vi "Host Save ID Data.vi"(11 "Input RY":T1) -> ()   [LabVIEW 2016]
uses:
  <vilib>/Utility/file.llb/Write Delimited Spreadsheet (string).vi
  <vilib>/Utility/file.llb/Write Delimited Spreadsheet (DBL).vi
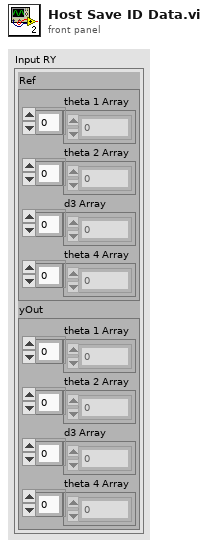
[diagram p1: front panel]
types:
  T1 = cluster{"Ref":cluster{"theta 1 Array":dbl[], "theta 2 Array":dbl[], "d3 Array":dbl[], "theta 4 Array":dbl[]}, "yOut":cluster{"theta 1 Array":dbl[], "theta 2 Array":dbl[], "d3 Array":dbl[], "theta 4 Array":dbl[]}}
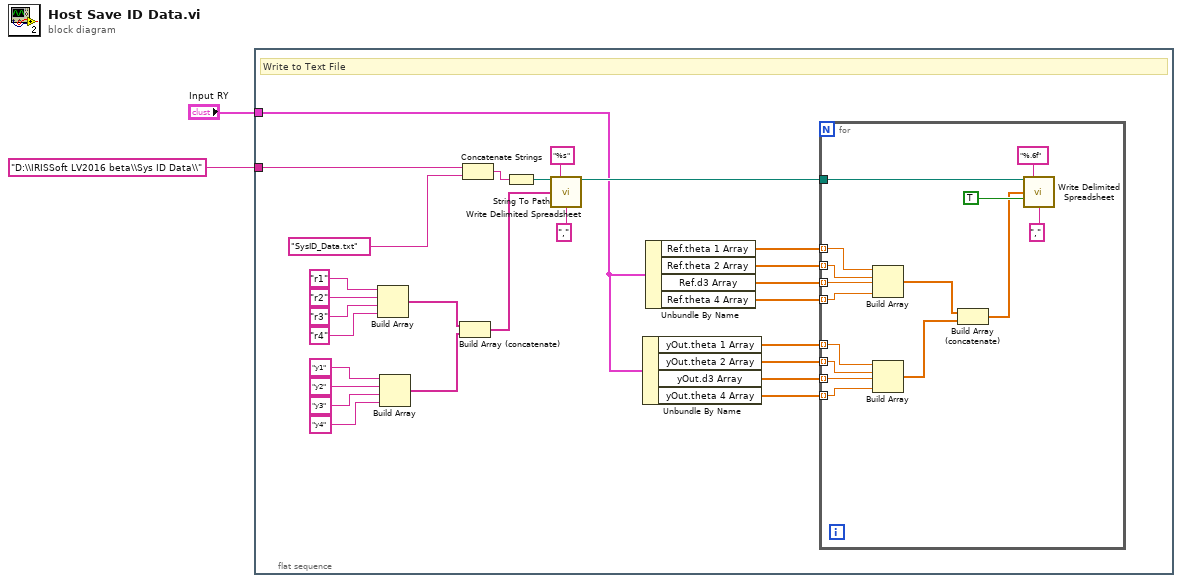
[diagram p0: block diagram]
diagram:
  n1 = flat-sequence {
    tunnel: "Input RY" -> [w13]
    tunnel: "D:\\IRISSoft LV2016 beta\\Sys ID Data\\" ("string") -> [w28]
    frame #0 {
      # "Write to Text File"
      n2 = Build Array("r1" ("string"), "r2" ("string"), "r3" ("string"), "r4" ("string")) -> (w4:string[])
      n3 = Build Array("y1" ("string"), "y2" ("string"), "y3" ("string"), "y4" ("string")) -> (w17:string[])
      n4 = Build Array (concatenate)(w4, w17) -> (w15:string[])
      n5 = Concatenate Strings(w28, "SysID_Data.txt" ("string")) -> (w29:string)
      n6 = String To Path(string=w29) -> (path=w27:path)
      n7 = call-poly <vilib>:"Write Delimited Spreadsheet.vi"("file path (dialog if empty)"=w27, "format (%s)"="%s" ("format (%.3f)"), "1D data"=w15, "delimiter (\\t)"="," ("delimiter (\\t)")) -> ("new file path (Not A Path if cancelled)"=w14:path)  [unwired: 10 in, 1 out]
      n8 = Unbundle By Name(w13) -> ("yOut.theta 1 Array"=w8:dbl[], "yOut.theta 2 Array"=w7:dbl[], "yOut.d3 Array"=w6:dbl[], "yOut.theta 4 Array"=w5:dbl[])
      n9 = Unbundle By Name(w13) -> ("Ref.theta 1 Array"=w12:dbl[], "Ref.theta 2 Array"=w11:dbl[], "Ref.d3 Array"=w10:dbl[], "Ref.theta 4 Array"=w9:dbl[])
      n10 = for {
        tunnel: w14 -> [w41]
        tunnel: w12 -> [w38] mode=indexing
        tunnel: w11 -> [w37] mode=indexing
        tunnel: w10 -> [w36] mode=indexing
        tunnel: w9 -> [w35] mode=indexing
        tunnel: w8 -> [w34] mode=indexing
        tunnel: w7 -> [w33] mode=indexing
        tunnel: w6 -> [w32] mode=indexing
        tunnel: w5 -> [w31] mode=indexing
        n11 = Build Array(w38, w37, w36, w35) -> (w39:dbl[])
        n12 = Build Array(w34, w33, w32, w31) -> (w40:dbl[])
        n13 = Build Array (concatenate)(w39, w40) -> (w30:dbl[])
        n14 = call-poly <vilib>:"Write Delimited Spreadsheet.vi"("file path (dialog if empty)"=w41, "format (%.3f)"="%.6f", "1D data"=w30, "append to file? (new file:F)"=TRUE, "delimiter (\\t)"="," ("delimiter (\\t)")) -> ()  [unwired: 9 in, 2 out]
      }
    }
  }
